vi "Set_Name Test.vi"(8 "error in (no error)":errorcluster caption="entrée d'erreur (pas d'erreur)", 10 "Name Test":string, 11 "Test (Default) en entrée":refnum<class "Test (Default).lvclass">) -> (0 "error out":errorcluster caption="sortie d'erreur", 3 "Test (Default) en sortie":refnum<class "Test (Default).lvclass">)   [LabVIEW 2020, in "Library Test.lvlib" / "Test (Default).lvclass"]
uses:
  Test (Default).lvclass
  Test (Default).lvclass/Test (Default).ctl
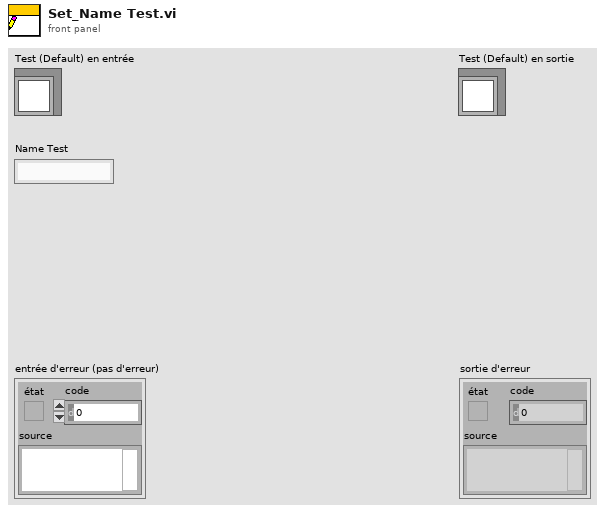
[diagram p1: front panel]
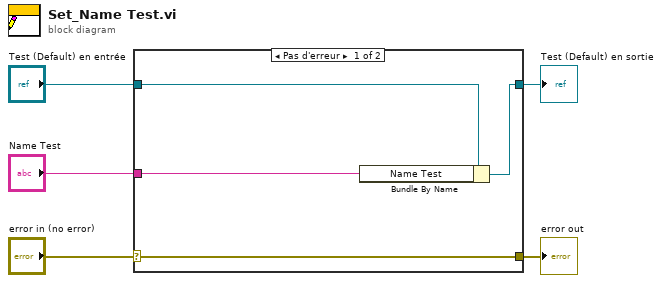
[diagram p0: block diagram]
diagram:
  n1 = case shown="Pas d'erreur" "error in (no error)" {
    selector: "error in (no error)" -> [w9 w10]
    tunnel: [w9 w10] -> w4
    tunnel: [w7 w11] -> w2
    tunnel: "Test (Default) en entrée" -> [w8 w11]
    tunnel: "Name Test" -> [w6 _]
    frame No Error {
      n2 = Bundle By Name(cluster=w8, "Name Test"=w6) -> (w7:refnum<class "Test (Default).lvclass">)
    }
    frame Error {
    }
  }
  "error out" <- w4
  "Test (Default) en sortie" <- w2
